vi "swag 1.vi"(1 "Temperatura °C":dbl) -> (0 "°Kelvin":dbl(slide) scale=-100.0..1000.0)   [LabVIEW 2014]
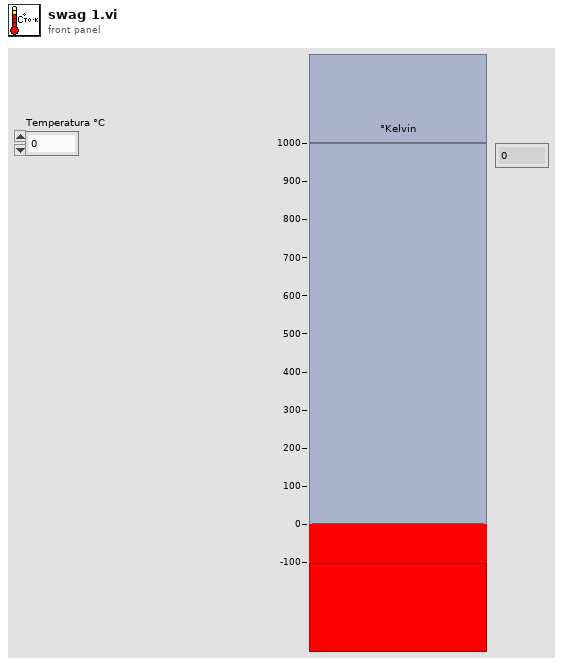
[diagram p1: front panel]
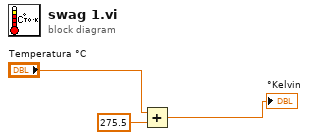
[diagram p0: block diagram]
diagram:
  n1 = Add(x="Temperatura °C", y=275.5) -> (x+y=→"°Kelvin":dbl)
